vi "Attenuation Control.vi"() -> ()   [LabVIEW 2021]
uses:
  <vilib>/Instr/_visa.llb/VISA Configure Serial Port (Instr).vi
panel:
  out "Logger":i32[](listbox)
  in  "log file path":path=path "M:/ECE480/log.csv"
  out "error out":errorcluster
  in  "Program Stop":bool
  in  "Program Start":bool
  in  "lower limit":u8
  in  "upper limit":u8
  out "CH4":u8(slide) scale=0.0..32.0
  out "CH3":u8(slide) scale=0.0..32.0
  out "CH2":u8(slide) scale=0.0..32.0
  out "CH1":u8(slide) scale=0.0..32.0
  in  "Channel 4":u8
  in  "Channel 3":u8
  in  "Channel 2":u8
  in  "Channel 1":u8
  in  "flow control (0:none)":u16(ring) items=["None", "XON/XOFF", "RTS/CTS", "XON/XOFF & RTS/CTS", "DTR/DSR", "XON/XOFF & DTR/DSR"]
  in  "stop bits (10: 1 bit)":u16(ring)=10 items=["1.0"=10, "1.5"=15, "2.0"=20]
  in  "timeout (10sec)":u32=10000
  in  "error in (no error)":errorcluster
  in  "parity (0:none)":enum16{"None", "Odd", "Even", "Mark", "Space"}(ring)
  in  "data bits (8)":u16=8 min=5 max=8 step=1
  in  "baud rate (9600)":u32=9600
  in  "VISA resource name":refnum<visa-resource-name>
  # "Channel Attenuation Display"
  # "USB Serial Port Configuration"
  # "Attenuation Limits"
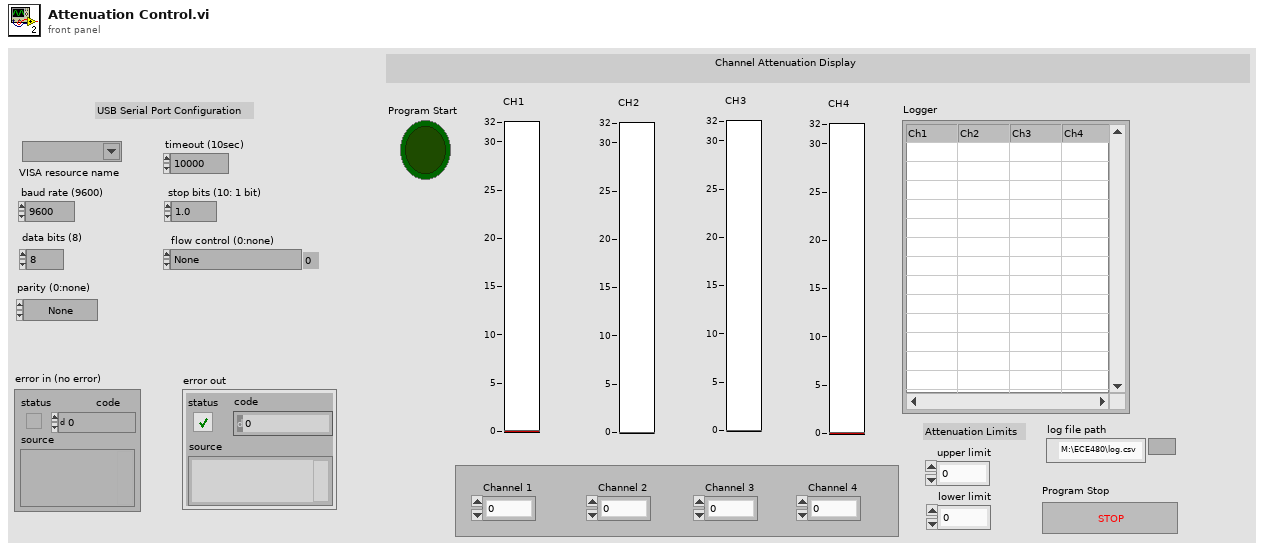
[diagram p1: front panel]
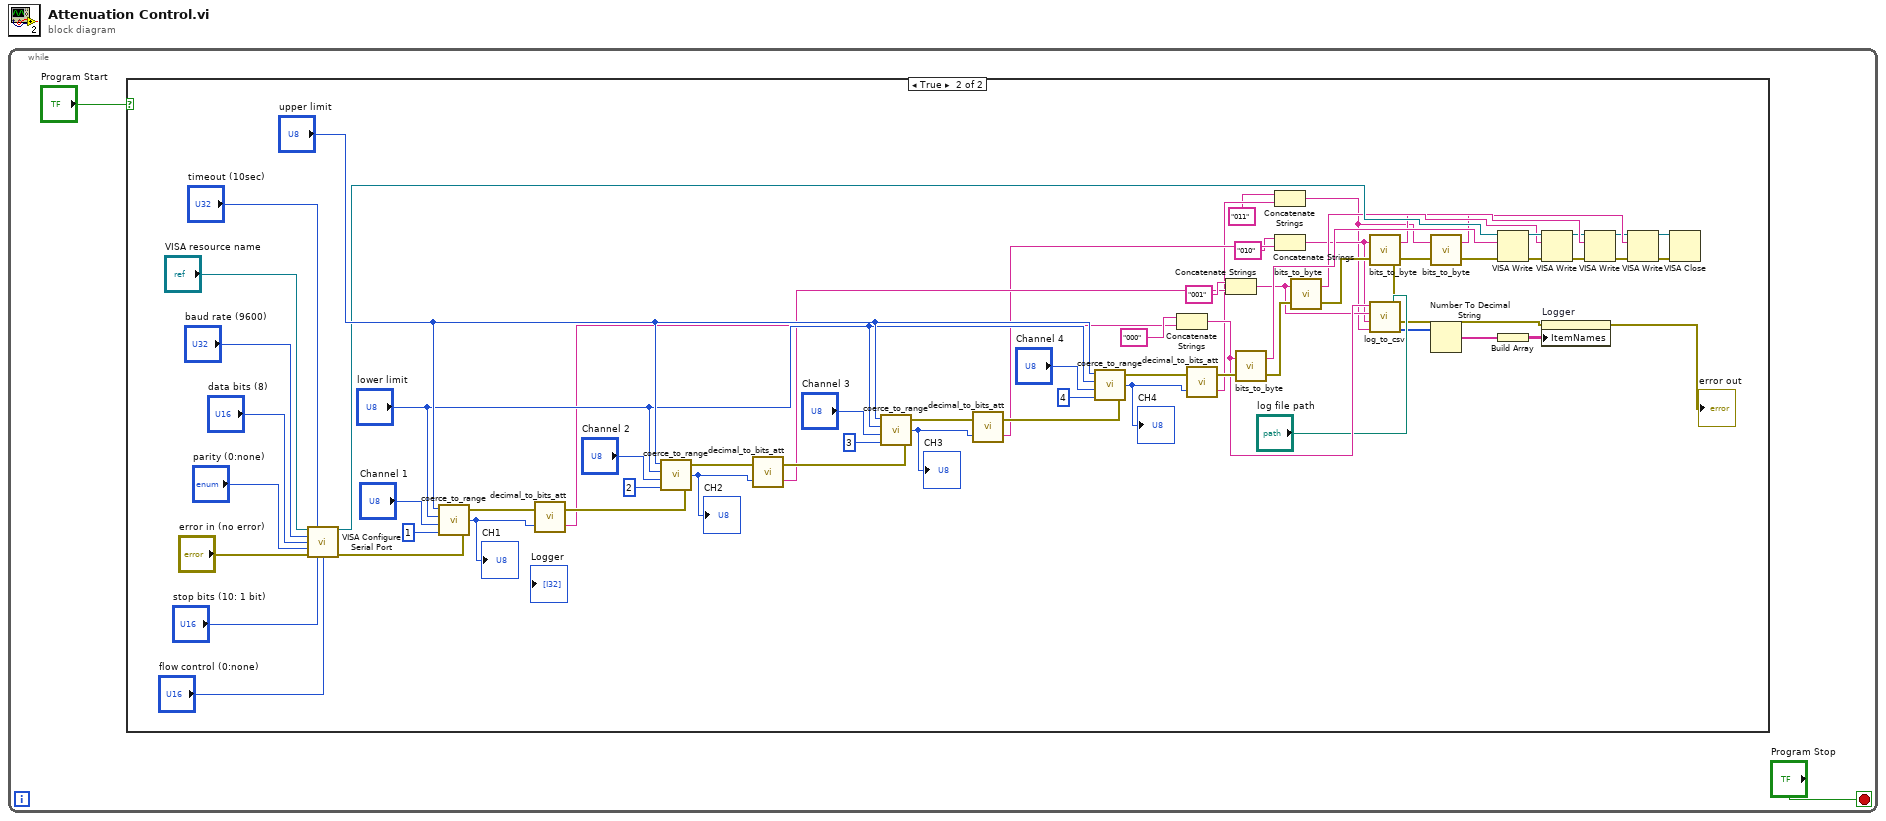
[diagram p0: block diagram]
diagram:
  n1 = while {
    stop <- "Program Stop" stop-if-true
    n2 = case shown="True" "Program Start" {
      frame False {
      }
      frame True {
        n3 = call-poly "VISA Configure Serial Port"("VISA resource name"="VISA resource name", "timeout (10sec)"="timeout (10sec)", "baud rate (9600)"="baud rate (9600)", "data bits (8)"="data bits (8)", "parity (0:none)"="parity (0:none)", "error in (no error)"="error in (no error)", "stop bits (10: 1 bit)"="stop bits (10: 1 bit)", "flow control (0:none)"="flow control (0:none)") -> ("VISA resource name out"=w35:refnum<visa-resource-name>, "error out"=w51:errorcluster)  [unwired: 6 in]
        n4 = call "coerce_to_range.vi"("error in (no error) 2"=w51, "channel no."=u8 1, "x"="Channel 1", "lower limit"="lower limit", "upper limit"="upper limit") -> ("coerced(x)"=w50:u8, "error in (no error)"=w46:errorcluster)
        "CH1" <- w50
        n5 = call "decimal_to_bits_att.vi"("attenuation decimal"=w50, "error in"=w46) -> ("attenuation binary"=w9:string, "error out"=w45:errorcluster)
        n6 = call "coerce_to_range.vi"("error in (no error) 2"=w45, "channel no."=u8 2, "x"="Channel 2", "lower limit"="lower limit", "upper limit"="upper limit") -> ("coerced(x)"=w49:u8, "error in (no error)"=w44:errorcluster)
        "CH2" <- w49
        n7 = call "decimal_to_bits_att.vi"("attenuation decimal"=w49, "error in"=w44) -> ("attenuation binary"=w7:string, "error out"=w43:errorcluster)
        n8 = call "coerce_to_range.vi"("error in (no error) 2"=w43, "channel no."=u8 3, "x"="Channel 3", "lower limit"="lower limit", "upper limit"="upper limit") -> ("coerced(x)"=w48:u8, "error in (no error)"=w42:errorcluster)
        "CH3" <- w48
        n9 = call "decimal_to_bits_att.vi"("attenuation decimal"=w48, "error in"=w42) -> ("attenuation binary"=w6:string, "error out"=w41:errorcluster)
        n10 = call "coerce_to_range.vi"("error in (no error) 2"=w41, "channel no."=u8 4, "x"="Channel 4", "lower limit"="lower limit", "upper limit"="upper limit") -> ("coerced(x)"=w47:u8, "error in (no error)"=w40:errorcluster)
        "CH4" <- w47
        n11 = Concatenate Strings("000" ("string"), w9) -> (w21:string)
        n12 = call "decimal_to_bits_att.vi"("attenuation decimal"=w47, "error in"=w40) -> ("attenuation binary"=w4:string, "error out"=w39:errorcluster)
        n13 = Concatenate Strings("001" ("string"), w7) -> (w20:string)
        n14 = call "bits_to_byte.vi"("error in"=w39, "Binary att & channel"=w21) -> ("error out"=w38:errorcluster, "Byte written out"=w34:string)
        n15 = Concatenate Strings("011" ("string"), w4) -> (w18:string)
        n16 = Concatenate Strings("010" ("string"), w6) -> (w19:string)
        n17 = call "bits_to_byte.vi"("error in"=w38, "Binary att & channel"=w20) -> ("error out"=w37:errorcluster, "Byte written out"=w31:string)
        n18 = call "bits_to_byte.vi"("error in"=w37, "Binary att & channel"=w19) -> ("error out"=w36:errorcluster, "Byte written out"=w30:string)
        n19 = call "bits_to_byte.vi"("error in"=w36, "Binary att & channel"=w18) -> ("error out"=w33:errorcluster, "Byte written out"=w29:string)
        n20 = VISA Write(VISA resource name=w35, write buffer=w34, error in (no error)=w33) -> (VISA resource name out=w32:refnum<visa-resource-name>, error out=w24:errorcluster)  [unwired: 1 out]
        n21 = VISA Write(VISA resource name=w32, write buffer=w31, error in (no error)=w24) -> (VISA resource name out=w26:refnum<visa-resource-name>, error out=w23:errorcluster)  [unwired: 1 out]
        n22 = VISA Write(VISA resource name=w26, write buffer=w30, error in (no error)=w23) -> (VISA resource name out=w25:refnum<visa-resource-name>, error out=w22:errorcluster)  [unwired: 1 out]
        n23 = VISA Write(VISA resource name=w25, write buffer=w29, error in (no error)=w22) -> (VISA resource name out=w28:refnum<visa-resource-name>, error out=w27:errorcluster)  [unwired: 1 out]
        n24 = VISA Close(VISA resource name=w28, error in (no error)=w27) -> (error out=w13:errorcluster)
        n25 = call "log_to_csv.vi"("error in"=w13, "log file path"="log file path", "channel 4 bit"=w18, "channel 3 bit"=w19, "channel 2 bit"=w20, "channel 1 bit"=w21) -> ("appended array"=w15:u8[], "error out"=w12:errorcluster)
        n26 = Number To Decimal String(number=w15) -> (decimal integer string=w16:string[])  [unwired: 1 in]
        n27 = Build Array(w16) -> (w14:string[][])
        n28 = property on="Logger" class="MCListbox (strict)"(error in=w12, "ItemNames"=w14) -> (error out=→"error out":errorcluster)  [unwired: 1 in, 1 out]
      }
    }
  }
